vi "ex_BackUpExistFileTDMS.vi"(8 "error in":errorcluster, 11 "file path":path) -> (0 "error out":errorcluster, 3 "dup file path":path)   [LabVIEW 2020]
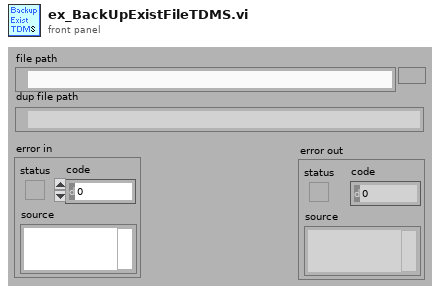
[diagram p1: front panel]
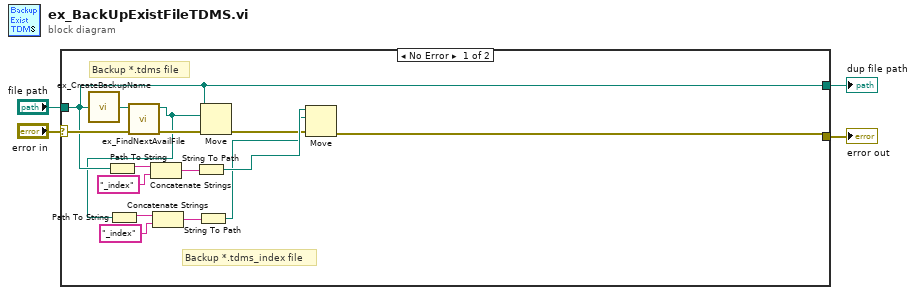
[diagram p0: block diagram]
diagram:
  n1 = case shown="No Error" "error in" {
    selector: "error in" -> [w19 w21]
    tunnel: [w5 w21] -> w3
    tunnel: "file path" -> [w10 w20]
    tunnel: [w10 w20] -> w1
    frame No Error {
      # "Backup *.tdms file"
      # "Backup *.tdms_index file"
      n2 = call "ex_CreateBackupName.vi"("original name"=w10) -> ("backup name"=w18:path)  [unwired: 4 out]
      n3 = Path To String(path=w10) -> (string=w16:string)
      n4 = call "ex_FindNextAvailFile.vi"("error in"=w19, "desired file path"=w18) -> ("error out"=w17:errorcluster, "next avail file path"=w9:path)  [unwired: 8 out]
      n5 = Path To String(path=w9) -> (string=w11:string)
      n6 = Concatenate Strings(w16, "_index" ("string")) -> (w14:string)
      n7 = Concatenate Strings(w11, "_index" ("string")) -> (w13:string)
      n8 = String To Path(string=w14) -> (path=w8:path)
      n9 = String To Path(string=w13) -> (path=w7:path)
      n10 = Move(source path=w10, error in=w17, 10:w9) -> (error out=w6:errorcluster)  [unwired: 4 out]
      n11 = Move(source path=w8, error in=w6, 10:w7) -> (error out=w5:errorcluster)  [unwired: 4 out]
    }
    frame Error {
    }
  }
  "error out" <- w3
  "dup file path" <- w1
